vi "Open.vi"(8 "error in (no error)":errorcluster, 11 "HAL in":refnum<class "HAL.lvclass">) -> (0 "error out":errorcluster, 3 "HAL out":refnum<class "HAL.lvclass">)   [LabVIEW 2019, in "Instrument.lvlib" / "HAL.lvclass"]
uses:
  HAL.lvclass
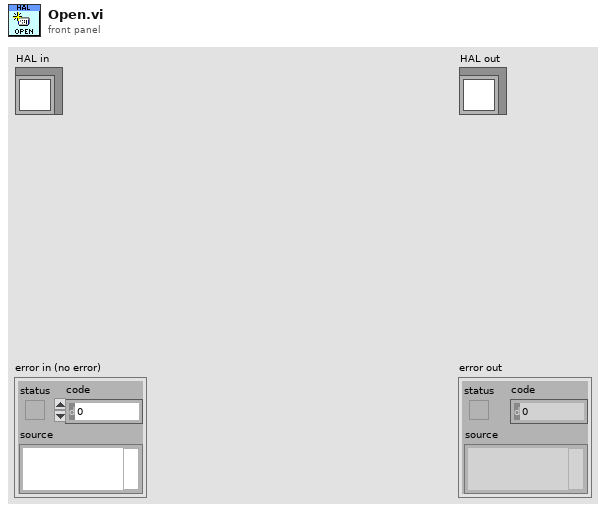
[diagram p1: front panel]
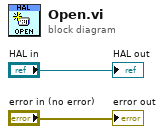
[diagram p0: block diagram]
diagram:
  "error out" <- "error in (no error)"
  "HAL out" <- "HAL in"
